vi "NI VeriStand - Remove Multiple Custom Device Items.vi"(7 "Skip action VI on delete (F)":bool, 8 "error in (no error)":errorcluster, 10 "Force Delete (F)":bool, 11 "Item Refs in":T1[](array[typedef]) format="%.0x") -> (0 "error out":errorcluster, 2 "Deleted?":bool)   [LabVIEW 2020, in "Custom Device API.lvlib"]
uses:
  <vilib>/NI VeriStand/Custom Device API/Custom Device API.lvlib
  <vilib>/NI VeriStand/Custom Device API/Custom Device Item Ref.ctl
  f2479363-73eb-461a-9b29-f8b0fabe25fc.vi
  <vilib>/NI VeriStand/Custom Device API/Custom Device Offline Path.vi
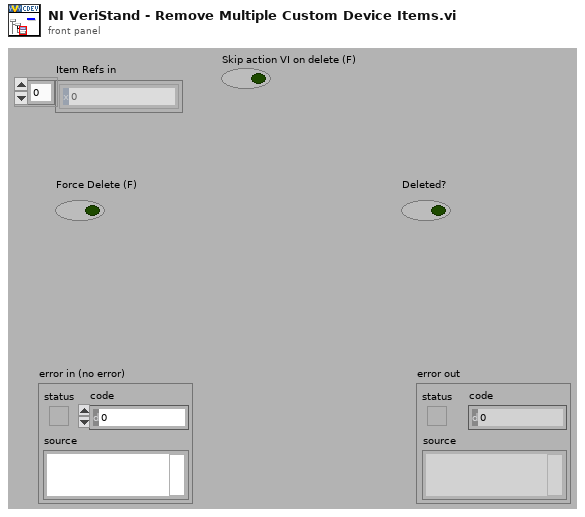
[diagram p1: front panel]
types:
  T1 = typedef "Custom Device API.lvlib/Custom Device Item Ref.ctl" = u64
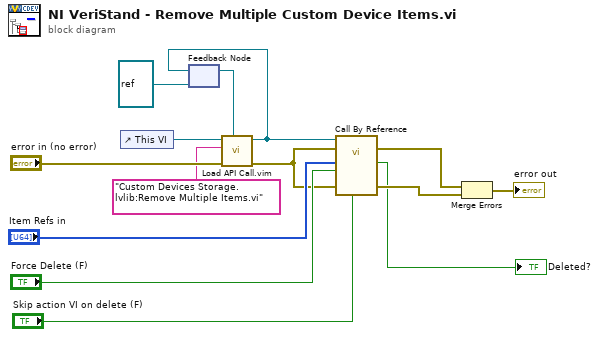
[diagram p0: block diagram]
diagram:
  n1 = control-ref of="This VI"() -> (w7:refnum<vi>)
  n2 = feedback #1(refnum<vi> refnum ("type specifier VI Refnum (for type only)")) -> (w8:refnum<vi>)
  n3 = call "Load API Call.vim"("VI reference in"=w8, "error in (no error)"="error in (no error)", "VI qualified name"="Custom Devices Storage.lvlib:Remove Multiple Items.vi", "Caller VI ref"=w7) -> ("error out"=w5:errorcluster, "VI reference"=w4:refnum<vi>)  [unwired: 6 in]
  n4 = feedback-in #1(w4) -> ()
  n5 = call-by-ref "?"(reference=w4, error in=w5, "Skip Action VI on Delete? (F)"="Skip action VI on delete (F)", 8:"error in (no error)"=w5, "Force Delete (F)"="Force Delete (F)", "Item Ref in"="Item Refs in") -> (error out=w1:errorcluster, 0:"error out"=w14:errorcluster, "Deleted?"=→"Deleted?":bool)  [unwired: 6 in, 1 out]
  n6 = Merge Errors(w1, w14) -> (→"error out":errorcluster)
